vi "运行demo守护脚本.vi"(8 "错误输入（无错误）":errorcluster) -> (0 "错误输出":errorcluster)   [LabVIEW 2016]
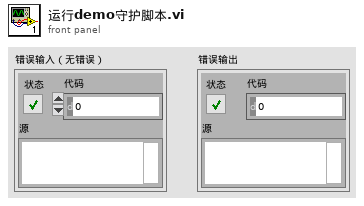
[diagram p1: front panel]
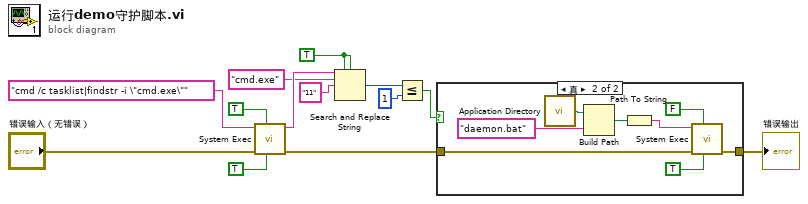
[diagram p0: block diagram]
diagram:
  w6 = TRUE ("替换全部？(F)")
  n1 = call <vilib>:"System Exec.vi"("run minimized? (F)"=TRUE, "wait until completion? (T)"=TRUE, "error in (no error)"="错误输入（无错误）", "command line"="cmd /c tasklist|findstr -i \"cmd.exe\"" ("字符串")) -> ("error out"=w3:errorcluster, "standard output"=w9:string)  [unwired: 4 in, 2 out]
  n2 = Search and Replace String(replace all?=w6, case sensitive?=w6, input string=w9, search string="cmd.exe" ("搜索字符串"), replace string="11" ("替换字符串(\"\")")) -> (number of replacements=w5:i32)  [unwired: 3 in, 3 out]
  n3 = Less Or Equal?(x=w5, y=1) -> (x <= y?=w2:bool)
  n4 = case shown="真" w2 {
    tunnel: w3 -> [w14 w17]
    tunnel: [w14 w16] -> w13
    frame False {
    }
    frame True {
      n5 = call <vilib>:"Application Directory.vi"() -> ("Application Directory"=w19:path)
      n6 = Build Path(base path=w19, name or relative path="daemon.bat" ("字符串")) -> (appended path=w18:path)
      n7 = Path To String(path=w18) -> (string=w21:string)
      n8 = call <vilib>:"System Exec.vi"("run minimized? (F)"=TRUE, "wait until completion? (T)"=FALSE, "error in (no error)"=w17, "command line"=w21) -> ("error out"=w16:errorcluster)  [unwired: 4 in, 3 out]
    }
  }
  "错误输出" <- w13
